vi "Read.vi"(8 "error in (no error)":errorcluster, 9 "timeout ms (5000)":i32=5000, 10 "# bytes to read":i32, 11 "dotNET SSL Socket in":refnum<class "dotNET SSL Socket.lvclass">) -> (0 "error out":errorcluster, 2 "Read Bytes":u8[](array[numeric]), 3 "dotNET SSL Socket out":refnum<class "dotNET SSL Socket.lvclass">)   [LabVIEW 2013, in "dotNET SSL Socket.lvlib" / "dotNET SSL Socket.lvclass"]
doc: "Reads data from a socket connection.\nWebSockets 2.0.0.30\nSam Sharp - MediaMongrels Ltd\nCopyright (c) 2019, MediaMongrels Ltd"
uses:
  dotNET SSL Socket.lvclass
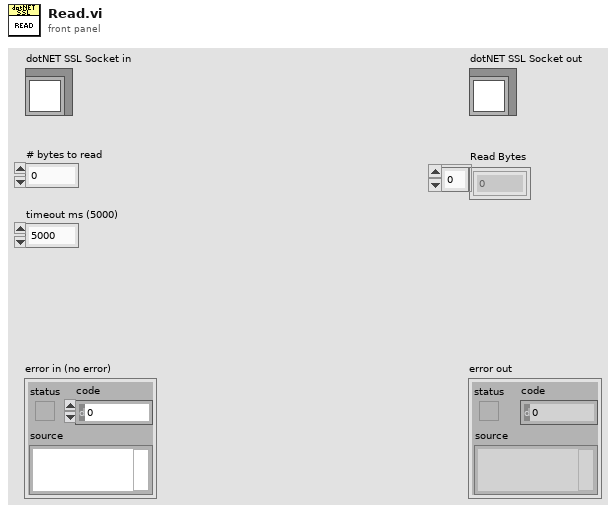
[diagram p1: front panel]
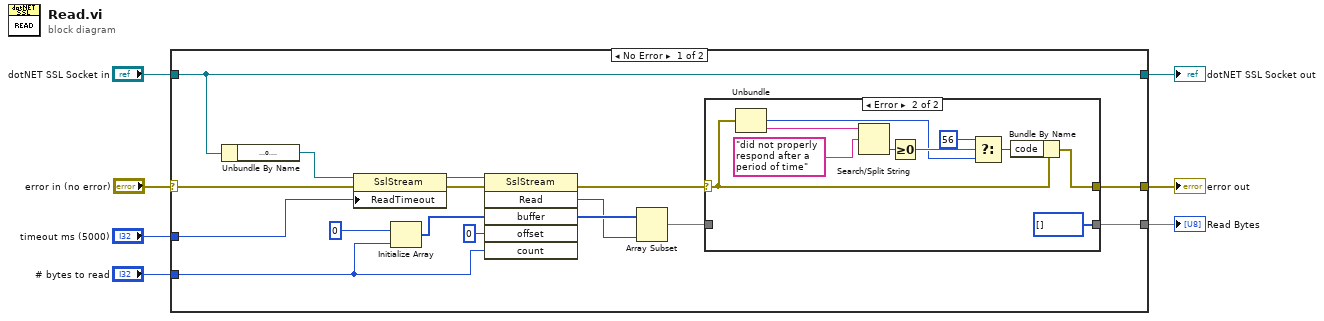
[diagram p0: block diagram]
diagram:
  n1 = case shown="No Error" "error in (no error)" {
    selector: "error in (no error)" -> [w9 w37]
    tunnel: "dotNET SSL Socket in" -> [w8 w36]
    tunnel: "timeout ms (5000)" -> [w20 _]
    tunnel: "# bytes to read" -> [w18 _]
    tunnel: [w12 w37] -> w4
    tunnel: [w11 _] -> w3
    tunnel: [w8 w36] -> w1
    frame No Error {
      n2 = Unbundle By Name(w8) -> ("SSLStream"=w23:refnum<k24>)
      n3 = property class="SslStream"(reference=w23, error in=w9, "ReadTimeout"=w20) -> (reference out=w22:refnum<k24>, error out=w21:errorcluster)
      n4 = Initialize Array(u8 0, w18) -> (w17:u8[])
      n5 = invoke class="SslStream" method="Read"(reference=w22, error in=w21, "buffer"=w17, "offset"=0, "count"=w18) -> (error out=w13:errorcluster, "Read"=w14:i32, "buffer"=w15:u8[])  [unwired: 1 in, 3 out]
      n6 = Array Subset(array=w15, length=w14) -> (w10:u8[])  [unwired: 1 in]
      n7 = case shown="Error" w13 {
        selector: w13 -> [w25 w31]
        tunnel: [w25 w29] -> w12
        tunnel: [w24 u8[] []] -> w11
        tunnel: w10 -> [w24 _]
        frame No Error {
        }
        frame Error {
          n8 = Unbundle(w31) -> ("code"=w28:i32, "source"=w35:string)  [unwired: 1 out]
          n9 = Search/Split String(string=w35, search string/char (-)="did not properly respond after a period of time") -> (offset of match=w33:i32)  [unwired: 1 in, 2 out]
          n10 = Greater Or Equal To 0?(x=w33) -> (x >= 0?=w32:bool)
          n11 = Select(t=56, s=w32, f=w28) -> (s? t:f=w30:i32)
          n12 = Bundle By Name(cluster=w31, "code"=w30) -> (w29:errorcluster)
        }
      }
    }
    frame Error {
    }
  }
  "error out" <- w4
  "dotNET SSL Socket out" <- w1
  "Read Bytes" <- w3
